vi "Open_file_set_refnum.vi"(8 "error in (no error)":errorcluster, 11 "DATA in":refnum<class "DATA.lvclass">) -> (0 "error out":errorcluster, 3 "DATA out":refnum<class "DATA.lvclass">)   [LabVIEW 2015, in "DATA.lvclass"]
uses:
  DATA.lvclass
  DATA.lvclass/DATA.ctl
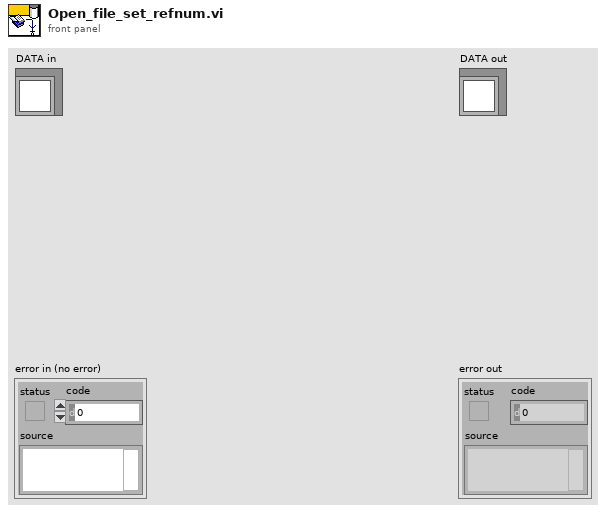
[diagram p1: front panel]
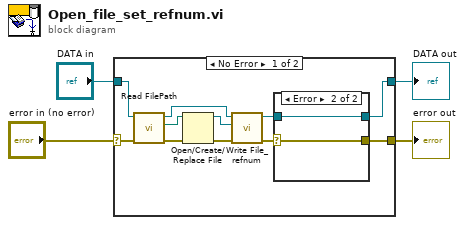
[diagram p0: block diagram]
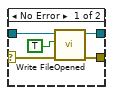
[diagram p2: hidden frame]
diagram:
  n1 = case shown="No Error" "error in (no error)" {
    selector: "error in (no error)" -> [w12 w24]
    tunnel: [w5 w24] -> w3
    tunnel: [w6 w23] -> w1
    tunnel: "DATA in" -> [w13 w23]
    frame No Error {
      n2 = call "Read FilePath.vi"("error in (no error)"=w12, "DATA in"=w13) -> ("error out"=w14:errorcluster, "FilePath"=w15:path, "DATA out"=w9:refnum<class "DATA.lvclass">)  [unwired: 7 in]
      n3 = Open/Create/Replace File(file path (use dialog)=w15, error in=w14) -> (refnum out=w11:refnum<file>, error out=w10:errorcluster)  [unwired: 4 in, 1 out]
      n4 = call "Write File_refnum.vi"("error in (no error)"=w10, "File_refnum"=w11, "DATA in"=w9) -> ("error out"=w7:errorcluster, "DATA out"=w8:refnum<class "DATA.lvclass">)  [unwired: 7 in]
      n5 = case shown="Error" w7 {
        selector: w7 -> [w18 w21]
        tunnel: w8 -> [w20 w22]
        tunnel: [w17 w22] -> w6
        tunnel: [w16 w21] -> w5
        frame No Error {
          n6 = call "Write FileOpened.vi"("error in (no error)"=w18, "FileOpened"=TRUE, "DATA in"=w20) -> ("error out"=w16:errorcluster, "DATA out"=w17:refnum<class "DATA.lvclass">)  [unwired: 7 in]
        }
        frame Error {
        }
      }
    }
    frame Error {
    }
  }
  "error out" <- w3
  "DATA out" <- w1
